vi "读线圈组.vi"(8 "error in":errorcluster, 10 "读多组线圈__输入":T1(array[cluster]), 11 "MB_实体":refnum<class "Modbus Master.lvclass">) -> (0 "输出簇":errorcluster, 2 "正在运行":bool, 3 "连接成功":bool)   [LabVIEW 2020]
uses:
  <vilib>/NI/Modbus Library/API/Master/Modbus Master.lvclass
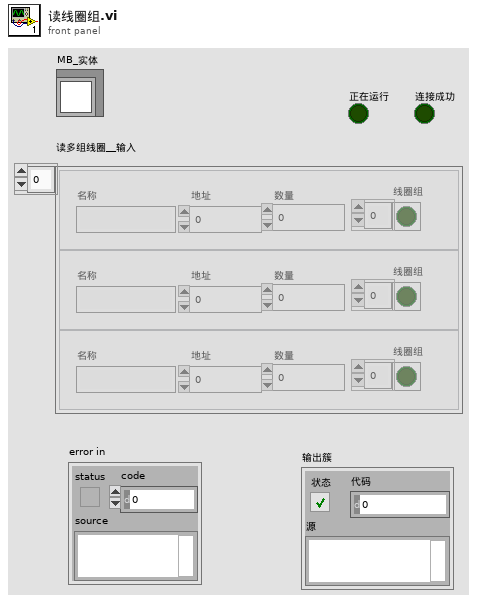
[diagram p1: front panel]
types:
  T1 = cluster{"地址":u16, "数量":u16, "名称":string, "线圈组":bool[]}[]
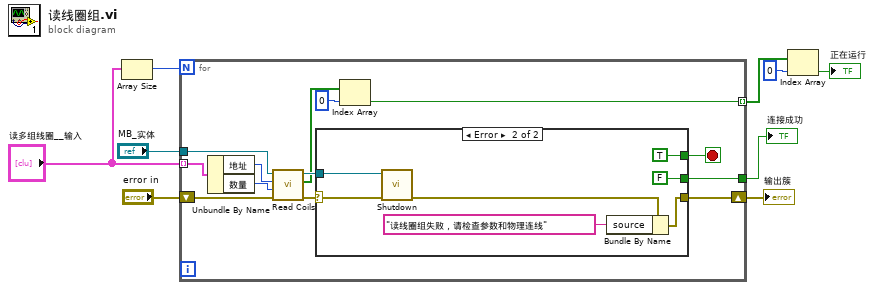
[diagram p0: block diagram]
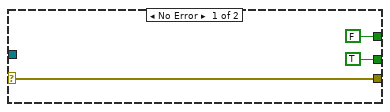
[diagram p2: hidden frame]
diagram:
  n1 = Array Size(array="读多组线圈__输入") -> (size(s)=w8:i32)
  n2 = for {
    N: w8 -> [_]
    tunnel: [w22] -> w6
    tunnel: "读多组线圈__输入" -> [w21] mode=indexing
    tunnel: [w10] -> w2 mode=indexing
    tunnel: "MB_实体" -> [w17]
    shift-right: [w14] -> w5
    shift-left: "error in" -> [w13]
    stop <- w20 stop-if-true
    n3 = Unbundle By Name(w21) -> ("地址"=w19:u16, "数量"=w18:u16)
    n4 = call-dynamic "Read Coils.vi"("error in"=w13, "number of inputs"=w18, "starting address"=w19, "Modbus master in"=w17) -> ("error out"=w15:errorcluster, "coils"=w12:bool[], "Modbus master out"=w16:refnum<class "Modbus Master.lvclass">)  [unwired: 5 in]
    n5 = case shown="Error" w15 {
      selector: w15 -> [w23 w30]
      tunnel: [TRUE FALSE] -> w22
      tunnel: [FALSE TRUE] -> w20
      tunnel: w16 -> [_ w29]
      tunnel: [w23 w26] -> w14
      frame No Error {
      }
      frame Error {
        n6 = call-dynamic "Shutdown.vi"("error in"=w30, "Modbus master in"=w29) -> ("error out"=w28:errorcluster)  [unwired: 9 in]
        n7 = Bundle By Name(cluster=w28, "source"="读线圈组失败，请检查参数和物理连线" ("消息")) -> (w26:errorcluster)
      }
    }
    n8 = Index Array(array=w12, index=0 ("索引")) -> (element=w10:bool)
  }
  "连接成功" <- w6
  "输出簇" <- w5
  n9 = Index Array(array=w2, index=0 ("索引")) -> (element=→"正在运行":bool)
